vi "Uninit.vi"(11 "MQTT-Client in":refnum<class "MQTT-Client.lvclass">) -> (3 "MQTT-Client out":refnum<class "MQTT-Client.lvclass">)   [LabVIEW 2023, in "MQTT-Client.lvlib" / "MQTT-Client.lvclass"]
doc: "This method is the inverse of the Pre Launch Init.vi. This method is called unconditionally at the end of an actor's lifetime, even if there was an error in Pre Launch Init.vi. Note that the self Enqueuer for the actor is already invalid by the time this VI executes: within this method, the actor may send messages to its caller but not to itself. This method executes before Last Ack is sent.\n\nThis method neither receives nor produces an error cluster. It is designed to provide an unconditional release of acquired resources. Any error raised during release is considered to be irrelevant to the actor's lifetime. If the actor truly needs to report some error status, it may send a message to caller or include information within itself that callers can examine when handling Last Ack."
uses:
  MQTT-Client.lvclass
  MQTT-Client.lvclass/MQTT-Client.ctl
  <vilib>/ActorFramework/Actor/Actor.lvclass
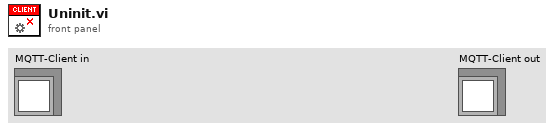
[diagram p1: front panel]
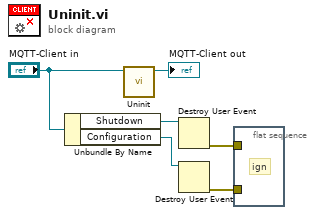
[diagram p0: block diagram]
diagram:
  n1 = Unbundle By Name("MQTT-Client in") -> ("Shutdown"=w5:refnum<user-event>, "Configuration"=w2:refnum<user-event>)
  n2 = call-parent "Uninit.vi"("Actor in"="MQTT-Client in") -> ("Actor out"=→"MQTT-Client out":refnum<class "MQTT-Client.lvclass">)  [unwired: 10 in]
  n3 = Destroy User Event(user event=w5) -> (error out=w4:errorcluster)  [unwired: 1 in]
  n4 = Destroy User Event(user event=w2) -> (error out=w1:errorcluster)  [unwired: 1 in]
  n5 = flat-sequence {
    tunnel: w4 -> [_]
    tunnel: w1 -> [_]
    frame #0 {
      # "ign"
    }
  }
